vi "Poll Event (OLD).vi"(8 "error in":errorcluster) -> (0 "error out":errorcluster, 1 "Event Data":u8[](array[numeric]), 2 "Event Type":u8, 3 "Return":i32)   [LabVIEW 2015]
doc: "Polls for currently pending events.\n\nIf event is not NULL, the next event is removed from the queue and stored in the SDL_Event structure pointed to by event.\n\nAs this function implicitly calls SDL_PumpEvents, you can only call this function in the thread that set the video mode.\n\nReturns 1 if there are any pending events, or 0 if there are none available."
uses:
  DLL/SDL2.dll
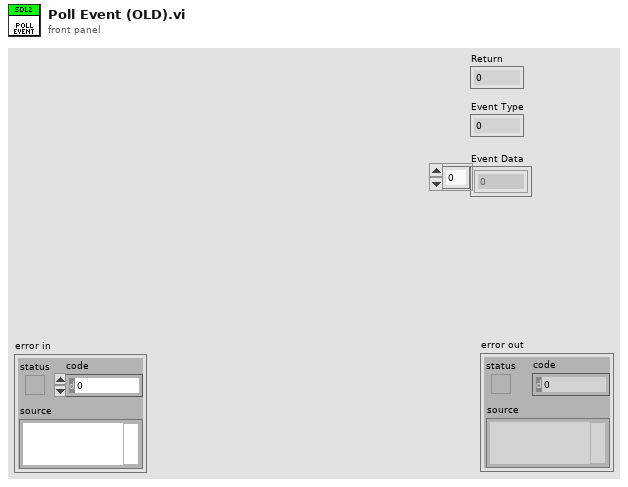
[diagram p1: front panel]
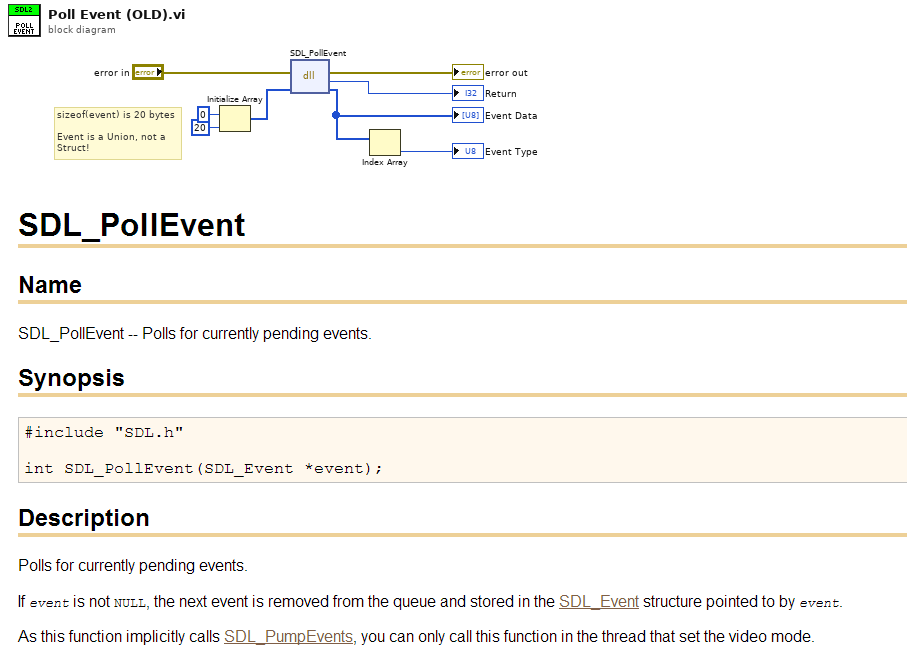
[diagram p0: block diagram]
diagram:
  # "sizeof(event) is 20 bytes\n\nEvent is a Union, not a Struct!"
  n1 = Initialize Array(u8 0, 20 ("dimension size")) -> (w3:u8[])
  n2 = dll-call lib="C:/dev/PGS/LabSDL2/Source/Libraries/LibSDL2 Wrapper/DLL/SDL2.dll" fn="SDL_PollEvent"(error in="error in", "event"=w3) -> (error out=→"error out":errorcluster, "return type"=→"Return":i32, "event"=w2:u8[])  [unwired: 2 in, 1 out]
  "Event Data" <- w2
  n3 = Index Array(array=w2) -> (element=→"Event Type":u8)  [unwired: 1 in]
